vi "Init.vi"(8 "error in (no error)":errorcluster, 11 "DynamicParameters in":refnum<class "DapperParameters.lvclass">) -> (0 "error out":errorcluster, 3 "DynamicParameters out":refnum<class "DapperParameters.lvclass">)   [LabVIEW 2020, in "ORM_Dapper.lvlib" / "DapperParameters.lvclass"]
uses:
  DapperParameters.lvclass
  DapperParameters.lvclass/DapperParameters.ctl
  C:/Viviota/Projects/R&D/LabVIEW_ORM/source/src/libraries/dapper/Dapper.dll
  libraries/dapper/Dapper.dll
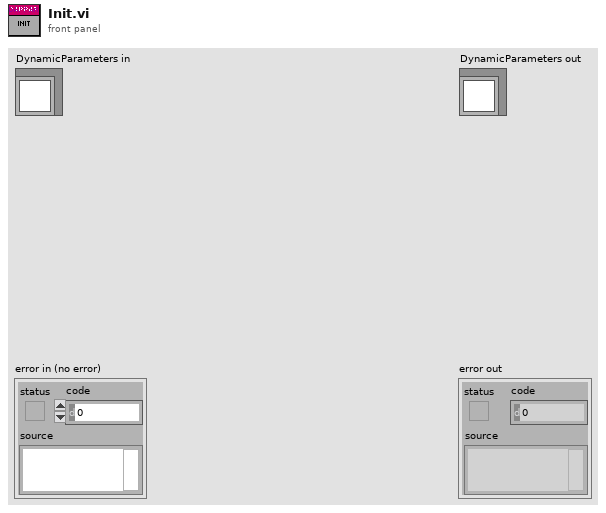
[diagram p1: front panel]
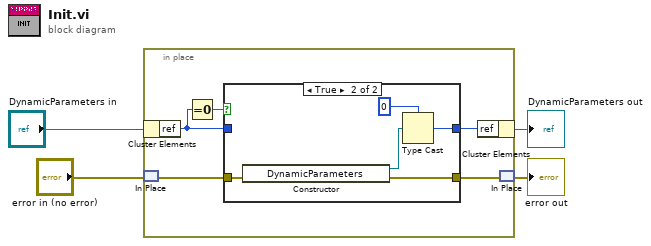
[diagram p0: block diagram]
diagram:
  n1 = in-place {
    n2 = in-place-cluster #1("DynamicParameters in") -> ("ref"=w7:u64)
    n3 = in-place-match #2("error in (no error)") -> (w9:errorcluster)
    n4 = Equal To 0?(x=w7) -> (x = 0?=w6:bool)
    n5 = case shown="True" w6 {
      tunnel: w9 -> [w10 w16]
      tunnel: [w10 w15] -> w8
      tunnel: [w11 w13] -> w5
      tunnel: w7 -> [w11 _]
      frame False {
      }
      frame True {
        n6 = constructor class="DynamicParameters"(error in=w16) -> (reference out=w14:refnum<k24>, error out=w15:errorcluster)  [unwired: 2 in, 1 out]
        n7 = Type Cast(type=u64 0 ("ref"), x=w14) -> (*(type *) &x=w13:u64)
      }
    }
    n8 = in-place-cluster #1("ref"=w5) -> (→"DynamicParameters out":refnum<class "DapperParameters.lvclass">)
    n9 = in-place-match #2(w8) -> (→"error out":errorcluster)
  }
